vi "P24LB-1.vi"() -> ()   [LabVIEW 2017]
uses:
  <vilib>/Instr/_visa.llb/VISA Configure Serial Port (Instr).vi
panel:
  out "String 2":string
  in  "stop":bool
  out "String":string
  in  "GIRO ANTIHORARIO":bool
  in  "VISA resource name":refnum<visa-resource-name>
  in  "GIRO HORARIO":bool
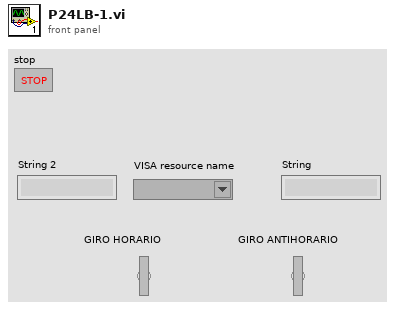
[diagram p1: front panel]
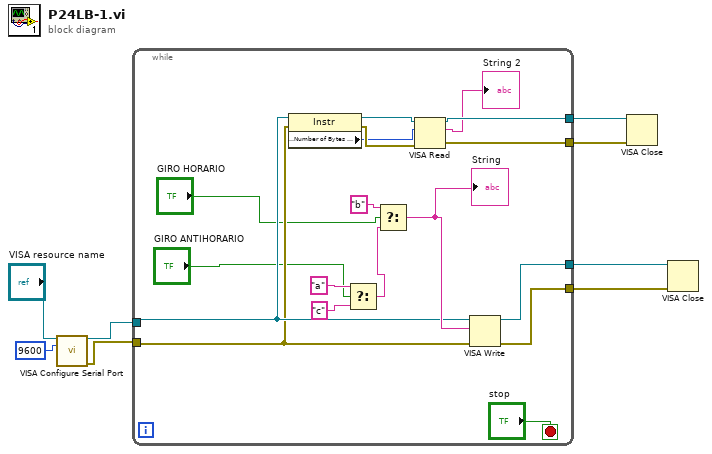
[diagram p0: block diagram]
diagram:
  n1 = call-poly "VISA Configure Serial Port"("VISA resource name"="VISA resource name", "baud rate (9600)"=u32 9600) -> ("VISA resource name out"=w6:refnum<visa-resource-name>, "error out"=w5:errorcluster)  [unwired: 12 in]
  n2 = while {
    tunnel: w6 -> [w13]
    tunnel: w5 -> [w12]
    tunnel: [w22] -> w4
    tunnel: [w21] -> w3
    tunnel: [w18] -> w2
    tunnel: [w17] -> w1
    stop <- "stop" stop-if-true
    n3 = property class="Instr"(reference=w13, error in=w12) -> (reference out=w16:refnum<visa-resource-name>, error out=w15:errorcluster, "Serial Settings:Number of Bytes at Serial Port"=w14:u32)
    n4 = Select(t="a", s="GIRO ANTIHORARIO", f="c") -> (s? t:f=w23:string)
    n5 = Select(t="b", s="GIRO HORARIO", f=w23) -> (s? t:f=w20:string)
    "String" <- w20
    n6 = VISA Read(VISA resource name=w16, byte count=w14, error in (no error)=w15) -> (VISA resource name out=w18:refnum<visa-resource-name>, read buffer=→"String 2":string, error out=w17:errorcluster)  [unwired: 1 out]
    n7 = VISA Write(VISA resource name=w13, write buffer=w20, error in (no error)=w12) -> (VISA resource name out=w21:refnum<visa-resource-name>, error out=w22:errorcluster)  [unwired: 1 out]
  }
  n8 = VISA Close(VISA resource name=w2, error in (no error)=w1) -> ()  [unwired: 1 out]
  n9 = VISA Close(VISA resource name=w3, error in (no error)=w4) -> ()  [unwired: 1 out]
